vi "告警信息解析.vi"(11 "告警信息":u16[](array[numeric]) caption="告警参数") -> ()   [LabVIEW 2016, in "数据传输系统-03.lvlib"]
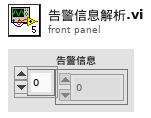
[diagram p1: front panel]
types:
  T1 = cluster{"告警信息[0]":u16, "告警信息[1]":u16, "告警信息[2]":u16, "告警信息[3]":u16, "告警信息[4]":u16, "告警信息[5]":u16}
  T2 = cluster{"告警信息[0]":bool, "告警信息[1]":bool, "告警信息[2]":bool, "告警信息[3]":bool, "告警信息[4]":bool, "告警信息[5]":bool}
  T3 = cluster{"setini":string, "sysini":string, "hechaini":string, "actualwrite":string, "actualread":string, "datasent":string, "反控命令信息队列":string, "反控与仪器交互":string}
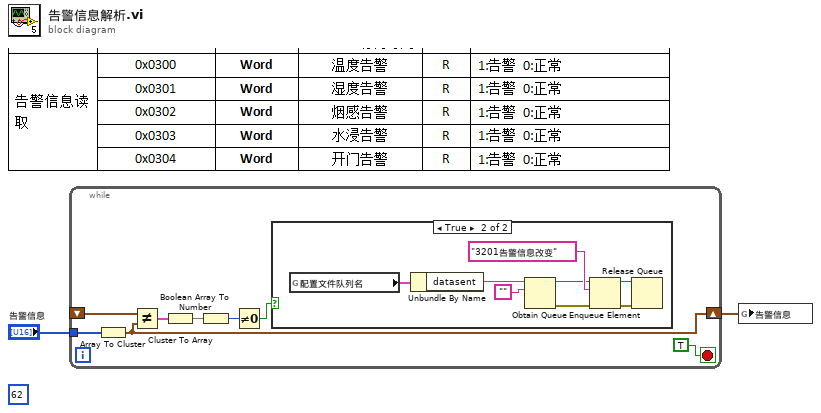
[diagram p0: block diagram]
diagram:
  (unwired) 62 ("索引")
  n1 = while {
    tunnel: "告警信息" -> [w9]
    shift-right: [w7] -> w1
    shift-left: _ -> [w8]
    stop <- TRUE stop-if-true
    n2 = Array To Cluster(array=w9) -> (cluster=w7:T1)
    n3 = Not Equal?(x=w8, y=w7) -> (x != y?=w5:T2)
    n4 = Cluster To Array(cluster=w5) -> (array=w4:bool[])
    n5 = Boolean Array To Number(Boolean array=w4) -> (number=w6:u32)
    n6 = Not Equal To 0?(x=w6) -> (x != 0?=w3:bool)
    n7 = case shown="True" w3 {
      frame False {
      }
      frame True {
        n8 = global read "全局1.vi" "配置文件队列名"() -> (w18:T3)
        n9 = Unbundle By Name(w18) -> ("datasent"=w11:string)
        n10 = Obtain Queue(name (unnamed)=w11, element data type="") -> (queue out=w13:refnum<queue>, error out=w15:errorcluster)  [unwired: 3 in, 1 out]
        n11 = Enqueue Element(queue=w13, element="3201告警信息改变" ("元素"), error in (no error)=w15) -> (queue out=w16:refnum<queue>, error out=w17:errorcluster)  [unwired: 1 in, 1 out]
        n12 = Release Queue(queue=w16, error in (no error)=w17) -> ()  [unwired: 1 in, 3 out]
      }
    }
  }
  n13 = global write "全局1.vi" "告警信息"(w1) -> ()
